vi "Error handler.vi"(8 "error indicator":errorcluster, 11 "error in":errorcluster) -> (0 "source out":string, 1 "code out":i32 format="%0.0f", 3 "error?":bool)   [LabVIEW 2020]
uses:
  <vilib>/Utility/error.llb/DialogType.ctl
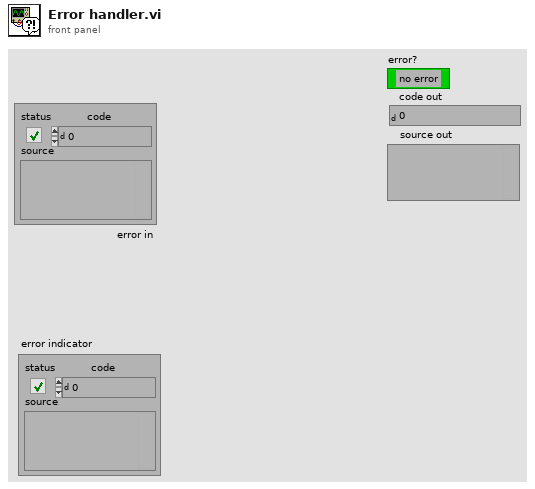
[diagram p1: front panel]
types:
  T1 = typedef "DialogType.ctl" = u16
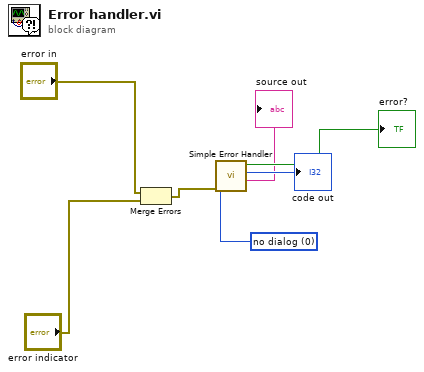
[diagram p0: block diagram]
diagram:
  w4 = T1 0 items=["no dialog", "OK message", "continue or stop message", "OK message + warnings", "continue/stop + warnings"] ("type of dialog (OK msg:1)")
  n1 = Merge Errors("error in", "error indicator") -> (w5:errorcluster)
  n2 = call <vilib>:"Simple Error Handler.vi"("type of dialog (OK msg:1)"=w4, "error in (no error)"=w5) -> ("error?"=→"error?":bool, "code out"=→"code out":i32, "source out"=→"source out":string)  [unwired: 3 in, 2 out]
